vi "Sierra - Frequency Drift test 2-26loop.vi"() -> ()   [LabVIEW 2015]
doc: "This VI demonstrates a simple procedure for setting up a spectrum analyzer, running an acquisition, and retrieving and plotting the waveform data.\n\nString indicators Binary WF Data and Sgl Float WF Data are initialized to empty strings. Waveform Graph is initialized to 0 for 100000 locations (just an arbitrary number for demonstration purposes).\n\ntkrsa6100 Initialize.vi opens the VISA Resource Name from the information entered by the user. It also presets the instrument by default to the Spectrum measurement. On completion it passes dup VISA Resource Name and error out to the following drivers.\n\nThe next VI to execute is tkrsa6100 Config Frequency.vi. Numeric control Center Freq (MHz)(50) is passed to the VI to set the center frequency to the default 50MHz value. The Set/Read Freq Setting (Set) is not wired since it defaults to SET, which is what is desired in this case. This is the case for all the configuration VI's in the example.\n\nThe next VI to execute is tkrsa6100 Config Spectrum Settings.vi. Enumerated control Spectrum Settings (CENTER FREQUENCY) is passed a Frequency Span constant and numeric control Freq Span (MHz) (40) to set the span to 40MHz.\n\nNext the reference level is set using tkrsa6100 Config RF Input.vi. Enumerated control Input Setting (REFERENCE LEVEL) is passed a Reference Level constant and numeric control Ref Level (dBm)(0) to set the reference level to 0dBm.\n\nNext the acquisition mode is set to single acquisition using tkrsa6100 Config Acquisition.vi. No parameters are passed since the default setting of this VI sets the acquisition mode to single.\n\nA single acquisition is then performed using tkrsa6100 Run Single Acquisition.vi. This VI sends an INIT command followed by a *OPC? Query. When the acquisition is completed the instrument returns a 1 and the next vi executes.\n\nThe binary waveform data is then retrieved by tkrsa6100 Spectrum Msmt Results.vi. The last acquisition data is retrieved by passing constant GET LAST ACQUISITION RESULT to enumerated input Run Acquisition and/or Get Result (RUN ACQUISITION & GET RESULT). The binary data is converted to a comma separated list of single precision floating point numbers by passing constant YES to enumerated input Convert Resp String (NO). The number of display points (total number of data bytes/4) is passed to a Spectral Display property node to scale the x axis of the graph. The binary data string from output Measurement Response String is copied to string indicator Binary WF Data. The converted binary data from output Converted Sgl Float Response String is copied to string indicator Sgl Float WF Data.\n\nSgl Float WF Data is then converted to an array by function Spreadsheet String to Array using a comma as the data separator. The output array is then passed to waveform graph Spectral Display for viewing.\n\nThe VISA Resource Name is closed using tkrsa6100 Close.vi."
panel:
  in  "Channel Selection":string(combo)
  out "Frequency at end of packet":dbl format="%#_15g"
  out "Drift between measurements":dbl
  out "Frequency at beginning of packet":dbl format="%#_15g"
  in  "VISA Resource Name":refnum<visa-resource-name>
  out "Sgl Float WF Data":string
  out "Binary WF Data":string
  out "Spectral Display":dbl[](graph)
  out "error out":errorcluster {"code" format="%#.0f"}
  # "RSA6106A/6114A Acquire and Fetch\nSpectral Analysis Display"
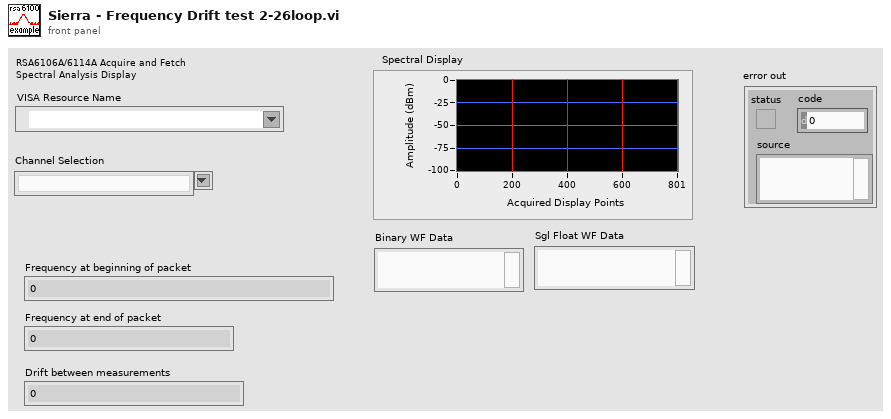
[diagram p1: front panel]
types:
  T1 = enum16{"CENTER FREQUENCY", "FREQUENCY SPAN", "RESOLUTION BW", "MAX REAL TIME SPAN (SET)", "START FREQUENCY", "STOP FREQUENCY", "FREQ STEP SIZE", "AUTO FREQ STEP ON", "AUTO FREQ STEP OFF", "AUTO RES BW ON", "AUTO RES BW OFF", "FFT WINDOW TYPE", "# POINTS", "RBW PROCESS ON", "RBW PROCESS OFF", "GAIN/BW OPTIMIZATION"}
  T2 = enum16{"RUN ACQUISITION  & GET RESULT", "GET LAST ACQUISITION RESULT"}
  T3 = enum16{"ANALYSIS REFERENCE", "ANALYSIS LENGTH", "ACTUAL ANALYSIS LENGTH (READ)", "AUTO ANALYSIS LENGTH ON", "AUTO ANALYSIS LENGTH OFF", "ANALYSIS OFFSET", "AUTO ANALYSIS OFFSET ON", "AUTO ANALYSIS OFFSET OFF", "SPECTRUM LENGTH", "ACTUAL SPECTRUM LENGTH (READ)", "AUTO SPECTRUM LENGTH ON", "AUTO SPECTRUM LENGTH OFF", "SPECTRUM OFFSET", "SPECTRUM TIME MODE", "DITHER MODE", "DITHER HW STATUS (READ)", "AUTO SPECTRUM OFFSETS AND ANALYSIS"}
  T4 = enum16{"TRIGGER SOURCE", "TRIGGER ON", "TRIGGER OFF", "TIME DELAY", "TIME POSITION", "TRIGGER EACH SEGMENT ON", "TRIGGER EACH SEGMENT OFF", "TRIGGER TYPE POWER", "TRIGGER TYPE FREQ MASK", "TRIGGER LEVEL", "TRIGGER SLOPE RISING", "TRIGGER SLOPE FALLING", "TDBW MODE ON", "TDBW MODE OFF", "TDBW", "ACTUAL TDBW (READ)", "CREATE NEW FMT (SET)", "SAVE FMT (SET)", "LOAD FMT (SET)", "FMT VIOLATION LOGIC", "FMT RBW AUTO", "FMT RBW MANUAL", "FMT RBW", "FORCE TRIGGER", "Trigger Position Auto"}
  T5 = enum16{"SPECTRUM ANALYZER", "DPSA", "SPECTROGRAM", "AMPL VS TIME", "FREQ VS TIME", "PHASE VS TIME", "IQ VS TIME", "TIME OVERVIEW"}
  T6 = enum16{"PEAK FIND (SET)", "NEXT PEAK LOWER (SET)", "NEXT PEAK HIGHER (SET)", "NEXT PEAK LEFT (SET)", "NEXT PEAK RIGHT (SET)", "MARKER TO CF (SET)", "MARKER TO TRACE", "MARKER FREQ", "MARKER AMPL (READ)", "DELTA MARKER FREQ (READ)", "DELTA MARKER AMPL (READ)"}
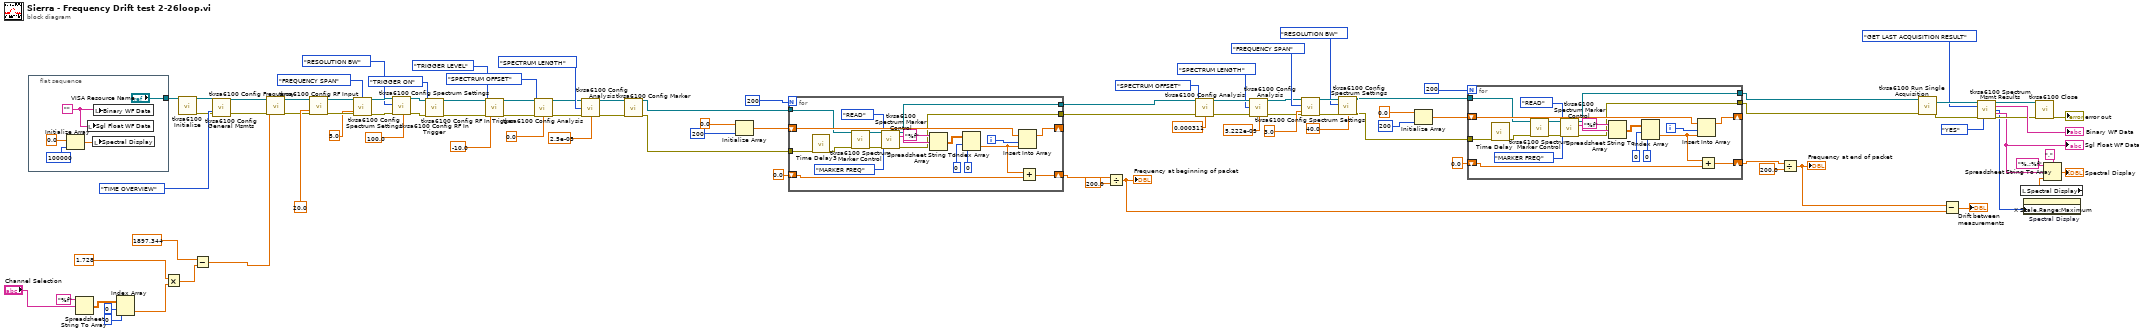
[diagram p0: block diagram]
diagram:
  n1 = flat-sequence {
    tunnel: ["VISA Resource Name"] -> w87
    frame #0 {
      w99 = ""
      n2 = Initialize Array(0.0 ("element"), 100000 ("dimension size")) -> (w101:dbl[])
      n3 = local write "Sgl Float WF Data"(w99) -> ()
      n4 = local write "Spectral Display"(w101) -> ()
      n5 = local write "Binary WF Data"(w99) -> ()
    }
  }
  n6 = Spreadsheet String To Array(format string="%f", spreadsheet string="Channel Selection") -> (array=w6:dbl[][])  [unwired: 2 in]
  n7 = Index Array(array=w6, index (row)=0, index (col)=0 ("disabled index (col)")) -> (element=w2:dbl)
  n8 = Multiply(x=1.728, y=w2) -> (x*y=w9:dbl)
  n9 = call <instrlib>:"tkrsa6100 Initialize.vi"("VISA Resource Name"=w87) -> ("dup VISA Resource Name"=w83:refnum<visa-resource-name>, "error out"=w84:errorcluster)  [unwired: 3 in, 10 out]
  n10 = Subtract(x=1897.344, y=w9) -> (x-y=w8:dbl)
  n11 = call <instrlib>:"tkrsa6100 Config General Msmts.vi"("VISA Resource Name"=w83, "Measurement\n(SPECTRUM ANALYZER)"=T5."TIME OVERVIEW" ("Measurement\n(SPECTRUM ANALYZER)"), "error in (no error)"=w84) -> ("dup VISA Resource Name"=w68:refnum<visa-resource-name>, "error out"=w67:errorcluster)  [unwired: 10 in, 1 out]
  n12 = call <instrlib>:"tkrsa6100 Config Frequency.vi"("VISA Resource Name"=w68, "Msmt Freq (MHz)\n(1000)"=w8, "error in (no error)"=w67) -> ("dup VISA Resource Name"=w66:refnum<visa-resource-name>, "error out"=w65:errorcluster)  [unwired: 1 in, 10 out]
  n13 = call <instrlib>:"tkrsa6100 Config RF Input.vi"("VISA Resource Name"=w66, "Ref Level (0)"=20.0 ("Ref Level (dBm)(0)"), "error in (no error)"=w65) -> ("dup VISA Resource Name"=w58:refnum<visa-resource-name>, "error out"=w57:errorcluster)  [unwired: 4 in, 7 out]
  n14 = call <instrlib>:"tkrsa6100 Config Spectrum Settings.vi"("VISA Resource Name"=w58, "Spectrum Settings\n (CENTER FREQUENCY)"=T1."FREQUENCY SPAN" ("Spectrum Settings\n (CENTER FREQUENCY)"), "Freq Span\n(MHz)(40)"=5.0 ("Freq Span\n(MHz)(40)"), "error in (no error)"=w57) -> ("dup VISA Resource Name"=w51:refnum<visa-resource-name>, "error out"=w50:errorcluster)  [unwired: 13 in, 1 out]
  n15 = call <instrlib>:"tkrsa6100 Config Spectrum Settings.vi"("VISA Resource Name"=w51, "Spectrum Settings\n (CENTER FREQUENCY)"=T1."RESOLUTION BW" ("Spectrum Settings\n (CENTER FREQUENCY)"), "error in (no error)"=w50, "Res BW (KHz)\n(300)"=100.0 ("Res BW (KHz)\n(300)")) -> ("dup VISA Resource Name"=w49:refnum<visa-resource-name>, "error out"=w48:errorcluster)  [unwired: 13 in, 1 out]
  n16 = call <instrlib>:"tkrsa6100 Config RF In Trigger.vi"("VISA Resource Name"=w49, "Trigger Settings\n(TRIGGER SOURCE)"=T4."TRIGGER ON" ("Trigger Settings\n(TRIGGER SOURCE)"), "error in (no error)"=w48) -> ("dup VISA Resource Name"=w73:refnum<visa-resource-name>, "error out"=w74:errorcluster)  [unwired: 14 in, 1 out]
  n17 = call <instrlib>:"tkrsa6100 Config RF In Trigger.vi"("VISA Resource Name"=w73, "Trigger Settings\n(TRIGGER SOURCE)"=T4."TRIGGER LEVEL" ("Trigger Settings\n(TRIGGER SOURCE)"), "error in (no error)"=w74, "Trig Level\n(dBm)(-10)"=-10.0 ("Trig Level (dBm)")) -> ("dup VISA Resource Name"=w54:refnum<visa-resource-name>, "error out"=w53:errorcluster)  [unwired: 13 in, 1 out]
  n18 = call <instrlib>:"tkrsa6100 Config Analysis.vi"("VISA Resource Name"=w54, "Analysis Setting\n(ANALYSIS REFERENCE)"=T3."SPECTRUM OFFSET" ("Analysis Setting\n(ANALYSIS REFERENCE)"), "error in (no error)"=w53, "Offset Tme (S)(0)"=0.0) -> ("dup VISA Resource Name"=w71:refnum<visa-resource-name>, "error out"=w72:errorcluster)  [unwired: 9 in, 1 out]
  n19 = call <instrlib>:"tkrsa6100 Config Analysis.vi"("VISA Resource Name"=w71, "Length (S)(0.022)"=2.5e-05, "Analysis Setting\n(ANALYSIS REFERENCE)"=T3."SPECTRUM LENGTH" ("Analysis Setting\n(ANALYSIS REFERENCE)"), "error in (no error)"=w72) -> ("dup VISA Resource Name"=w45:refnum<visa-resource-name>, "error out"=w44:errorcluster)  [unwired: 9 in, 1 out]
  n20 = call <instrlib>:"tkrsa6100 Config Marker.vi"("VISA Resource Name"=w45, "error in (no error)"=w44) -> ("dup VISA Resource Name"=w31:refnum<visa-resource-name>, "error out"=w30:errorcluster)  [unwired: 11 in, 1 out]
  n21 = Initialize Array(0.0 ("element"), 200 ("dimension size")) -> (w32:dbl[])
  n22 = for {
    N: 200 ("Numeric") -> [_]
    shift-right: [w114] -> _
    shift-left: w32 -> [w113]
    tunnel: [w106] -> w28
    tunnel: [w109] -> w29
    tunnel: w31 -> [w108]
    tunnel: w30 -> [w107]
    shift-right: [w104] -> w27
    shift-left: 0.0 -> [w103]
    i -> [w112]
    n23 = call "Time Delay3"("error in (no error)"=w107) -> ("error out"=w116:errorcluster)  [unwired: 10 in]
    n24 = call <instrlib>:"tkrsa6100 Spectrum Marker Control.vi"("VISA Resource Name"=w108, "error in (no error)"=w116) -> ("dup VISA Resource Name"=w122:refnum<visa-resource-name>, "error out"=w115:errorcluster)  [unwired: 11 in, 1 out]
    n25 = call <instrlib>:"tkrsa6100 Spectrum Marker Control.vi"("VISA Resource Name"=w122, "Set/Read\nMarker Functions (SET)"=enum16{"SET", "READ"}."READ" ("Set/Read\nMarker Functions (SET)"), "Marker Function\n(PEAK FIND)"=T6."MARKER FREQ" ("Marker Function\n(PEAK FIND)"), "error in (no error)"=w115) -> ("dup VISA Resource Name"=w106:refnum<visa-resource-name>, "Marker\nResponse String"=w121:string, "error out"=w109:errorcluster)  [unwired: 9 in]
    n26 = Spreadsheet String To Array(format string="%f", spreadsheet string=w121) -> (array=w119:dbl[][])  [unwired: 2 in]
    n27 = Index Array(array=w119, index (row)=0, index (col)=0 ("disabled index (col)")) -> (element=w105:dbl)
    n28 = Insert Into Array(array=w113, index=w112, new element=w105) -> (w114:dbl[])
    n29 = Add(x=w105, y=w103) -> (x+y=w104:dbl)
  }
  n30 = Divide(x=w27, y=200.0) -> (x/y=w19:dbl)
  "Frequency at beginning of packet" <- w19
  n31 = call <instrlib>:"tkrsa6100 Config Analysis.vi"("VISA Resource Name"=w28, "Analysis Setting\n(ANALYSIS REFERENCE)"=T3."SPECTRUM OFFSET" ("Analysis Setting\n(ANALYSIS REFERENCE)"), "error in (no error)"=w29, "Offset Tme (S)(0)"=0.000311) -> ("dup VISA Resource Name"=w62:refnum<visa-resource-name>, "error out"=w61:errorcluster)  [unwired: 9 in, 1 out]
  n32 = call <instrlib>:"tkrsa6100 Config Analysis.vi"("VISA Resource Name"=w62, "Length (S)(0.022)"=5.222e-05, "Analysis Setting\n(ANALYSIS REFERENCE)"=T3."SPECTRUM LENGTH" ("Analysis Setting\n(ANALYSIS REFERENCE)"), "error in (no error)"=w61) -> ("dup VISA Resource Name"=w37:refnum<visa-resource-name>, "error out"=w36:errorcluster)  [unwired: 9 in, 1 out]
  n33 = call <instrlib>:"tkrsa6100 Config Spectrum Settings.vi"("VISA Resource Name"=w37, "Spectrum Settings\n (CENTER FREQUENCY)"=T1."FREQUENCY SPAN" ("Spectrum Settings\n (CENTER FREQUENCY)"), "Freq Span\n(MHz)(40)"=3.0 ("Freq Span\n(MHz)(40)"), "error in (no error)"=w36) -> ("dup VISA Resource Name"=w41:refnum<visa-resource-name>, "error out"=w40:errorcluster)  [unwired: 13 in, 1 out]
  n34 = call <instrlib>:"tkrsa6100 Config Spectrum Settings.vi"("VISA Resource Name"=w41, "Spectrum Settings\n (CENTER FREQUENCY)"=T1."RESOLUTION BW" ("Spectrum Settings\n (CENTER FREQUENCY)"), "error in (no error)"=w40, "Res BW (KHz)\n(300)"=40.0 ("Res BW (KHz)\n(300)")) -> ("dup VISA Resource Name"=w21:refnum<visa-resource-name>, "error out"=w20:errorcluster)  [unwired: 13 in, 1 out]
  n35 = Initialize Array(0.0 ("element"), 200 ("dimension size")) -> (w22:dbl[])
  n36 = for {
    N: 200 ("Numeric") -> [_]
    shift-right: [w134] -> _
    shift-left: w22 -> [w133]
    tunnel: [w126] -> w17
    tunnel: [w129] -> w16
    tunnel: w21 -> [w128]
    tunnel: w20 -> [w127]
    shift-right: [w124] -> w14
    shift-left: 0.0 -> [w123]
    i -> [w132]
    n37 = call "Time Delay"("error in (no error)"=w127) -> ("error out"=w136:errorcluster)  [unwired: 10 in]
    n38 = call <instrlib>:"tkrsa6100 Spectrum Marker Control.vi"("VISA Resource Name"=w128, "error in (no error)"=w136) -> ("dup VISA Resource Name"=w142:refnum<visa-resource-name>, "error out"=w135:errorcluster)  [unwired: 11 in, 1 out]
    n39 = call <instrlib>:"tkrsa6100 Spectrum Marker Control.vi"("VISA Resource Name"=w142, "Set/Read\nMarker Functions (SET)"=enum16{"SET", "READ"}."READ" ("Set/Read\nMarker Functions (SET)"), "Marker Function\n(PEAK FIND)"=T6."MARKER FREQ" ("Marker Function\n(PEAK FIND)"), "error in (no error)"=w135) -> ("dup VISA Resource Name"=w126:refnum<visa-resource-name>, "Marker\nResponse String"=w141:string, "error out"=w129:errorcluster)  [unwired: 9 in]
    n40 = Spreadsheet String To Array(format string="%f", spreadsheet string=w141) -> (array=w139:dbl[][])  [unwired: 2 in]
    n41 = Index Array(array=w139, index (row)=0, index (col)=0 ("disabled index (col)")) -> (element=w125:dbl)
    n42 = Insert Into Array(array=w133, index=w132, new element=w125) -> (w134:dbl[])
    n43 = Add(x=w125, y=w123) -> (x+y=w124:dbl)
  }
  n44 = Divide(x=w14, y=200.0) -> (x/y=w13:dbl)
  "Frequency at end of packet" <- w13
  n45 = call <instrlib>:"tkrsa6100 Run Single Acquisition.vi"("VISA Resource Name"=w17, "error in (no error)"=w16) -> ("dup VISA Resource Name"=w76:refnum<visa-resource-name>, "error out"=w75:errorcluster)  [unwired: 12 out]
  n46 = Subtract(x=w13, y=w19) -> (x-y=→"Drift between measurements":dbl)
  n47 = call <instrlib>:"tkrsa6100 Spectrum Msmt Results.vi"("VISA Resource Name"=w76, "Run Acquisition and/or \nGet Result (RUN ACQUISITION & GET RESULT)"=T2."GET LAST ACQUISITION RESULT" ("Run Acquisition and/or \nGet Result (RUN ACQUISITION & GET RESULT)"), "error in (no error)"=w75, "Convert Resp\nString(NO)"=enum16{"NO", "YES"}."YES" ("Convert Resp\nString(NO)")) -> ("dup VISA Resource Name"=w90:refnum<visa-resource-name>, "Measurement\nResponse String"=→"Binary WF Data":string, "# Data Points"=w88:i32, "Converted Sgl Float\nResponse String"=w89:string, "error out"=w92:errorcluster)  [unwired: 7 in]
  "Sgl Float WF Data" <- w89
  n48 = local read "Spectral Display"() -> (w97:dbl[])
  n49 = property on="Spectral Display" class="WFGraph (strict)"("X Scale.Range:Maximum"=w88) -> ()  [unwired: 2 in, 2 out]
  n50 = call <instrlib>:"tkrsa6100 Close.vi"("VISA Resource Name"=w90, "error in (no error)"=w92) -> ("error out"=→"error out":errorcluster)  [unwired: 13 out]
  n51 = Spreadsheet String To Array(delimiter (Tab)=",", format string="%.;%f", spreadsheet string=w89, array type (2D Dbl)=w97) -> (array=→"Spectral Display":dbl[])
